vi "SaveConfig.vi"(8 "error in (no error)":errorcluster, 11 "Camera_Prime95B in":refnum<class "Camera_Prime95B.lvclass">) -> (0 "error out":errorcluster, 3 "Camera_Prime95B out":refnum<class "Camera_Prime95B.lvclass">)   [LabVIEW 2020, in "Camera_Prime95B.lvlib" / "Camera_Prime95B.lvclass"]
uses:
  Camera_Prime95B.lvclass
  Hardware Abstraction Layer/Component/Camera/Camera/Camera.lvclass
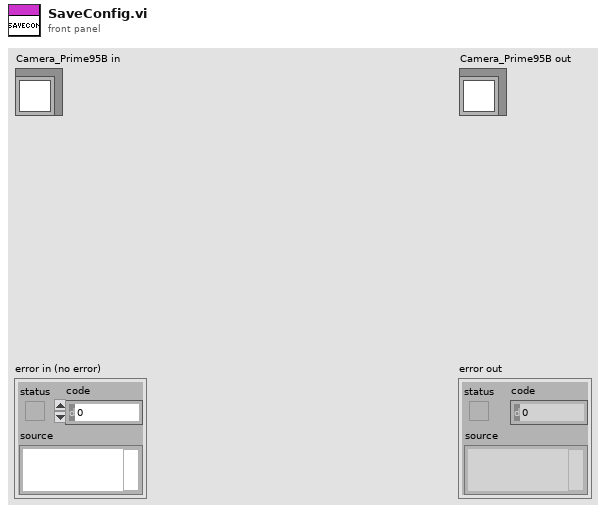
[diagram p1: front panel]
types:
  T1 = typedef "NI_LVConfig.lvlib/Config Data RefNum.ctl" = refnum<k1>
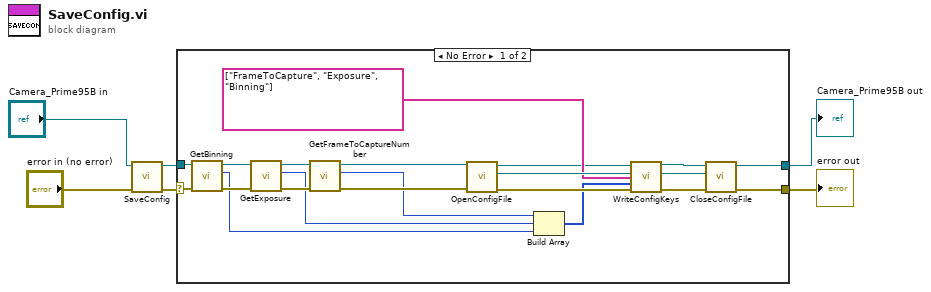
[diagram p0: block diagram]
diagram:
  n1 = call-parent "SaveConfig.vi"("error in (no error)"="error in (no error)", "GRMActor in"="Camera_Prime95B in") -> ("error out"=w3:errorcluster, "GRMActor out"=w4:refnum<class "Camera_Prime95B.lvclass">)  [unwired: 8 in]
  n2 = case shown="No Error" w3 {
    selector: w3 -> [w27 w28]
    tunnel: [w24 w28] -> w1
    tunnel: [w22 w29] -> w2
    tunnel: w4 -> [w12 w29]
    frame No Error {
      n3 = call-dynamic "GetBinning.vi"("error in (no error)"=w27, "Camera in"=w12) -> ("error out"=w13:errorcluster, "Setting.Binning.BinX"=w10:i32, "Camera out"=w11:refnum<class "Camera_Prime95B.lvclass">)  [unwired: 6 in, 1 out]
      n4 = call-dynamic "GetExposure.vi"("error in (no error)"=w13, "Camera in"=w11) -> ("error out"=w15:errorcluster, "Setting.Exposure"=w9:i32, "Camera out"=w14:refnum<class "Camera_Prime95B.lvclass">)  [unwired: 7 in]
      n5 = call-dynamic "GetFrameToCaptureNumber.vi"("error in (no error)"=w15, "Camera in"=w14) -> ("error out"=w17:errorcluster, "Setting.FramesToCapture"=w8:i32, "Camera out"=w16:refnum<class "Camera_Prime95B.lvclass">)  [unwired: 7 in]
      n6 = call-dynamic "OpenConfigFile.vi"("error in (no error)"=w17, "GRMActor in"=w16) -> ("error out"=w25:errorcluster, "refnum"=w21:T1, "GRMActor out"=w18:refnum<class "Camera_Prime95B.lvclass">)  [unwired: 7 in]
      n7 = Build Array(w8, w9, w10) -> (w7:i32[])
      n8 = call-dynamic "WriteConfigKeys.vi"("GRMActor in"=w18, "Config Refnum"=w21, "Keys"=string[] ["FrameToCapture", "Exposure", "Binning"] ("Values"), "IntValue"=w7, "error in (no error)"=w25) -> ("GRMActor out"=w23:refnum<class "Camera_Prime95B.lvclass">, "Config Refnum dup"=w20:T1, "error out"=w26:errorcluster)  [unwired: 8 in]
      n9 = call-dynamic "CloseConfigFile.vi"("error in (no error)"=w26, "refnum"=w20, "GRMActor in"=w23) -> ("error out"=w24:errorcluster, "GRMActor out"=w22:refnum<class "Camera_Prime95B.lvclass">)  [unwired: 7 in]
    }
    frame Error {
    }
  }
  "error out" <- w1
  "Camera_Prime95B out" <- w2
